vi "InitialStateNode_Create.vi"(0 "reference":refnum<class "InitialStateNode.lvclass">, 5 "error in (no error)":errorcluster, 6 "GoopReferenceIn":T1) -> (14 "reference out":refnum<class "InitialStateNode.lvclass">, 16 "# of objects":i32, 19 "error out":errorcluster)   [LabVIEW 2012, in "InitialStateNode.lvclass"]
doc: "Creates and initializes a new InitialStateNode object.\n\nThis object should be destroyed using a InitialStateNode destructor VI or a virtual base class destructor VI.\n\n[GOOP 2.1]"
uses:
  <resource>/Framework/Providers/Open_GDS/UML/InitialStateNode_class/InitialStateNode.lvclass
  <resource>/Framework/Providers/Open_GDS/UML/AbstractNode_class/ObjectReference.ctl
  <resource>/Framework/Providers/Open_GDS/UML/MultiLineString_class/SizeType.ctl
  <resource>/Framework/Providers/Open_GDS/UML/General/Rectangle/Rectangle Rectangle2D.ctl
  <resource>/Framework/Providers/Open_GDS/UML/MultiLineString_class/JustificationType.ctl
  <resource>/Framework/Providers/Open_GDS/UML/MultiLineString_class/MultiLineString.lvclass
  <resource>/Framework/Providers/Open_GDS/UML/RectangularNode_class/RectangularNode.lvclass
  <resource>/Framework/Providers/Open_GDS/UML/AbstractNode_class/AbstractNode.lvclass
panel:
  # "The input reference should only\nbe wired when this method is called\nby a sub class constructor."
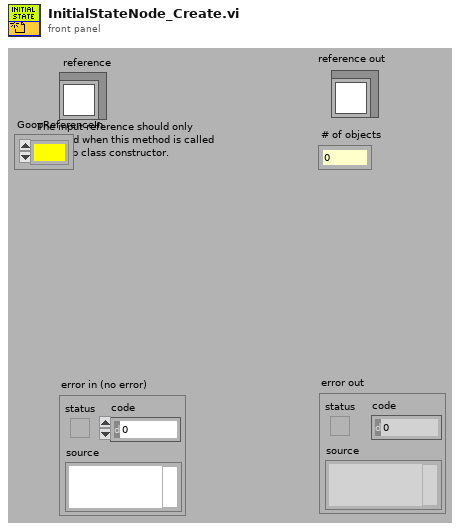
[diagram p1: front panel]
types:
  T1 = typedef "AbstractNode.lvclass/ObjectReference.ctl" = refnum<k1>
  T2 = typedef "MultiLineString.lvclass/JustificationType.ctl" = enum16{"LEFT", "CENTER", "RIGHT"}
  T3 = typedef "Rectangle Rectangle2D.ctl" = cluster{"x":dbl, "y":dbl, "width":dbl, "height":dbl}
  T4 = typedef "MultiLineString.lvclass/SizeType.ctl" = enum16{"LARGE", "NORMAL", "SMALL"}
  T5 = typedef "InitialStateNode.lvclass/ObjectAttributes.ctl" = cluster{"Base class":T6, "name":refnum<class "MultiLineString.lvclass">, "DEFAULT_WIDTH":i32, "DEFAULT_HEIGHT":i32}
  T6 = typedef "RectangularNode.lvclass/ObjectAttributes.ctl" = cluster{"Base class":T7, "bounds":T3}
  T7 = typedef "AbstractNode.lvclass/ObjectAttributes.ctl" = cluster{"parent":refnum<class "AbstractNode.lvclass">, "children":refnum<class "AbstractNode.lvclass">[], "Hidden":bool}
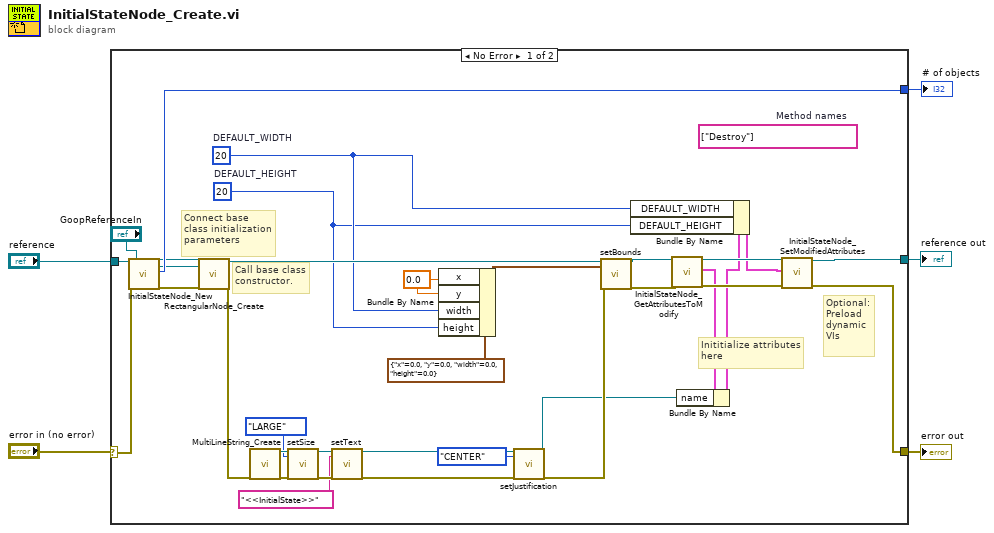
[diagram p0: block diagram]
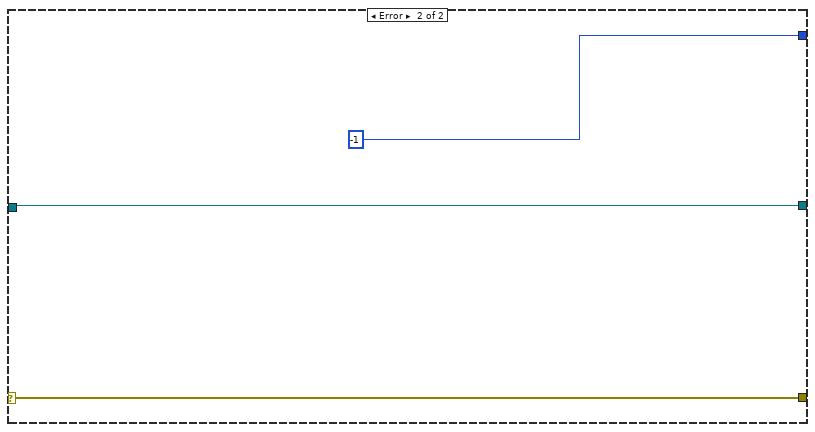
[diagram p2: hidden frame]
diagram:
  n1 = case shown="No Error" "error in (no error)" {
    selector: "error in (no error)" -> [w39 w41]
    tunnel: [w34 w40] -> w5
    tunnel: [w33 w41] -> w4
    tunnel: [w38 -1 ("Nr of open handles")] -> w3
    tunnel: "reference" -> [w37 w40]
    frame No Error {
      w23 = 0.0 ("x")
      (unwired) string[] ["Destroy"]  # Method names
      w20 = 20  # DEFAULT_HEIGHT
      w22 = 20  # DEFAULT_WIDTH
      # "Connect base\nclass initialization\nparameters"
      # "Call base class\nconstructor."
      # "Optional:\nPreload\ndynamic\nVIs"
      # "Inititialize attributes\nhere"
      n2 = call <resource>:"InitialStateNode_New.vi"("reference in"=w37, "error in (no error)"=w39, "GoopReferenceIn"="GoopReferenceIn") -> ("GoopReferenceOut"=w7:T1, "reference out"=w19:refnum<class "InitialStateNode.lvclass">, "# of objects"=w38:i32, "error out"=w32:errorcluster)  [unwired: 2 in, 11 out]
      n3 = call <resource>:"RectangularNode_Create.vi"("reference"=w19, "error in (no error)"=w32, "GoopReferenceIn"=w7) -> ("reference out"=w26:refnum<class "InitialStateNode.lvclass">, "error out"=w31:errorcluster)  [unwired: 15 out]
      n4 = call <resource>:"MultiLineString_Create.vi"("error in (no error)"=w31) -> ("reference out"=w30:refnum<class "MultiLineString.lvclass">, "error out"=w29:errorcluster)  [unwired: 3 in, 14 out]
      n5 = call <resource>:"setSize.vi"("reference"=w30, "size"=SizeType."LARGE", "error in (no error)"=w29) -> ("reference out"=w16:refnum<class "MultiLineString.lvclass">, "error out"=w15:errorcluster)  [unwired: 15 out]
      n6 = call-dynamic "setText.vi"("reference"=w16, "text"="<<InitialState>>", "error in (no error)"=w15) -> ("reference out"=w10:refnum<class "MultiLineString.lvclass">, "error out"=w11:errorcluster)  [unwired: 15 in]
      n7 = Bundle By Name(cluster=T3 {"x"=0.0, "y"=0.0, "width"=0.0, "height"=0.0} ("bounds"), "x"=w23, "y"=w23, "width"=w22, "height"=w20) -> (w25:T3)
      n8 = call <resource>:"setJustification.vi"("reference"=w10, "justification"=JustificationType."CENTER", "error in (no error)"=w11) -> ("reference out"=w9:refnum<class "MultiLineString.lvclass">, "error out"=w21:errorcluster)  [unwired: 15 out]
      n9 = call-dynamic "setBounds.vi"("reference"=w26, "bounds"=w25, "error in (no error)"=w21) -> ("reference out"=w6:refnum<class "InitialStateNode.lvclass">, "error out"=w17:errorcluster)  [unwired: 15 in]
      n10 = call <resource>:"InitialStateNode_GetAttributesToModify.vi"("reference in"=w6, "error in (no error)"=w17) -> ("reference out"=w35:refnum<class "InitialStateNode.lvclass">, "Attributes"=w18:T5, "error out"=w36:errorcluster)  [unwired: 1 in, 14 out]
      n11 = Bundle By Name(cluster=w18, "name"=w9) -> (w13:T5)
      n12 = Bundle By Name(cluster=w13, "DEFAULT_WIDTH"=w22, "DEFAULT_HEIGHT"=w20) -> (w12:T5)
      n13 = call <resource>:"InitialStateNode_SetModifiedAttributes.vi"("reference in"=w35, "Attributes"=w12, "error in (no error)"=w36) -> ("reference out"=w34:refnum<class "InitialStateNode.lvclass">, "error out"=w33:errorcluster)  [unwired: 3 in, 12 out]
    }
    frame Error {
    }
  }
  "error out" <- w4
  "reference out" <- w5
  "# of objects" <- w3
